vi "Newport ITX-D3N Data Filter.vi"(7 "iTHX Commands":T2="*SRTF", 8 "Error In":errorcluster, 11 "Current Data":dbl) -> (0 "Error Out":errorcluster, 2 "In Range?":bool, 3 "Data Output":dbl)   [LabVIEW 2023]
uses:
  Type Definitions/iTHX.ctl
  Type Definitions/iBTHX.ctl
panel:
  in  "iBTHX":T1="*SRH2"
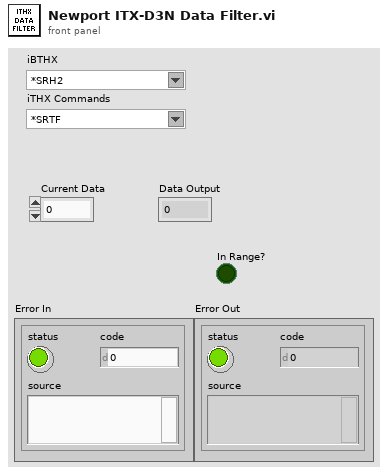
[diagram p1: front panel]
types:
  T1 = typedef "iBTHX.ctl" = string
  T2 = typedef "iTHX.ctl" = string
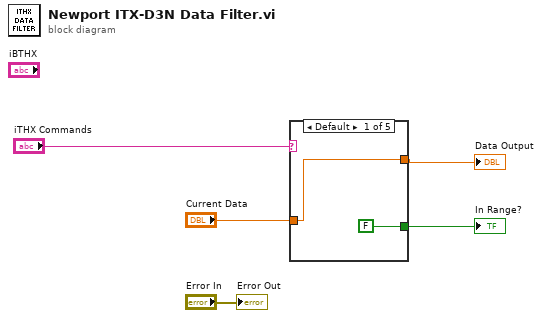
[diagram p0: block diagram]
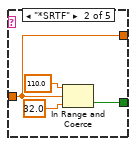
[diagram p2: hidden frame]
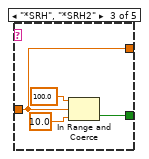
[diagram p3: hidden frame]
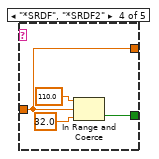
[diagram p4: hidden frame]
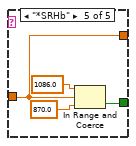
[diagram p5: hidden frame]
diagram:
  n1 = case shown="Default" "iTHX Commands" {
    tunnel: "Current Data" -> [w7 w8 w12 w16 w20]
    tunnel: [w7 w8 w12 w16 w20] -> w1
    tunnel: [FALSE w9 w15 w17 w21] -> w3
    frame Default {
    }
    frame "*SRTF" {
      n2 = In Range and Coerce(upper limit=110.0, x=w8, lower limit=32.0) -> (In Range?=w9:bool)  [unwired: 1 out]
    }
    frame "*SRH", "*SRH2" {
      n3 = In Range and Coerce(upper limit=100.0, x=w12, lower limit=10.0) -> (In Range?=w15:bool)  [unwired: 1 out]
    }
    frame "*SRDF", "*SRDF2" {
      n4 = In Range and Coerce(upper limit=110.0, x=w16, lower limit=32.0) -> (In Range?=w17:bool)  [unwired: 1 out]
    }
    frame "*SRHb" {
      n5 = In Range and Coerce(upper limit=1086.0, x=w20, lower limit=870.0) -> (In Range?=w21:bool)  [unwired: 1 out]
    }
  }
  "Data Output" <- w1
  "In Range?" <- w3
  "Error Out" <- "Error In"
